vi "Set Scroll Vis.vi"(8 "error in (no error)":errorcluster, 10 "Scroll Visible":bool, 11 "ArrayManager in":refnum<class "ArrayManager.lvclass">) -> (0 "error out":errorcluster, 3 "ArrayManager out":refnum<class "ArrayManager.lvclass">)   [LabVIEW 2020, in "OOPanel.lvlib" / "ArrayManager.lvclass"]
uses:
  <vilib>/IlluminatedG/IG OOPanel/OOPanel/ArrayManager/ArrayManager.lvclass
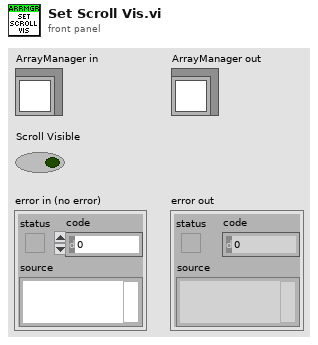
[diagram p1: front panel]
types:
  T1 = typedef "OOPanel.lvlib/ArrayManager.lvclass/UI Refs.ctl" = cluster{"SubPanels":refnum<vi>[], "Scrollbar":refnum<vi>, "Panel VI":refnum<vi>, "Container":refnum<vi>}
  T2 = typedef "OOPanel.lvlib/ArrayManager.lvclass/State Ref.ctl" = cluster{"Running":bool, "Borders":bool, "Total Height":dbl, "Scroll Visible":bool, "Background":u32}
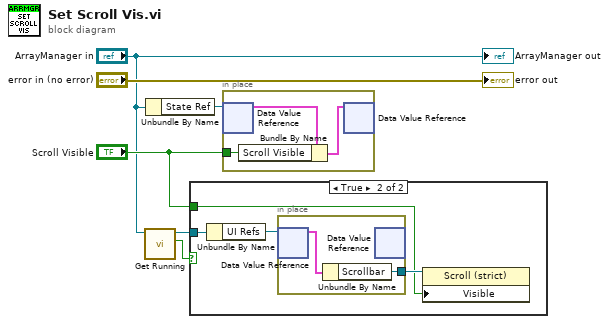
[diagram p0: block diagram]
diagram:
  n1 = call <vilib>:"Get Running.vi"("ArrayManager in"="ArrayManager in") -> ("Running"=w1:bool, "ArrayManager out"=w2:refnum<class "ArrayManager.lvclass">)  [unwired: 8 in, 1 out]
  n2 = Unbundle By Name("ArrayManager in") -> ("State Ref"=w5:refnum<data-value>)
  n3 = case shown="True" w1 {
    tunnel: "Scroll Visible" -> [_ w9]
    tunnel: w2 -> [_ w8]
    frame False {
    }
    frame True {
      n4 = Unbundle By Name(w8) -> ("UI Refs"=w7:refnum<data-value>)
      n5 = in-place {
        in-place-border: [w11] -> w10
        n6 = in-place-dvr #1(w7) -> (w12:T1)  [unwired: 1 out]
        n7 = Unbundle By Name(w12) -> ("Scrollbar"=w11:refnum<vi>)
        n8 = in-place-dvr #1() -> ()  [unwired: 1 in, 2 out]
      }
      n9 = property class="Scroll (strict)"(reference=w10, "Visible"=w9) -> ()  [unwired: 1 in, 2 out]
    }
  }
  n10 = in-place {
    in-place-border: "Scroll Visible" -> [w13]
    n11 = in-place-dvr #2(w5) -> (w15:T2)  [unwired: 1 out]
    n12 = Bundle By Name(cluster=w15, "Scroll Visible"=w13) -> (w14:T2)
    n13 = in-place-dvr #2(w14) -> ()  [unwired: 2 out]
  }
  "error out" <- "error in (no error)"
  "ArrayManager out" <- "ArrayManager in"
